vi "Filter Get Mode.vi"(11 "mode":u32) -> (2 "function return":u32, 3 "mode out":u32)   [LabVIEW 2018, in "AndorSDK.lvlib"]
doc: "EXPNETTYPE unsigned int WINAPI Filter_GetMode(unsigned int * mode);"
uses:
  AndorSDK.lvlib
  ATMCD32D.dll
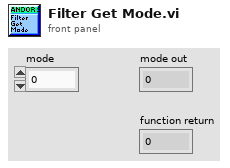
[diagram p1: front panel]
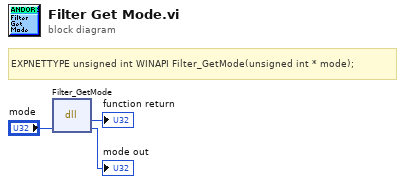
[diagram p0: block diagram]
diagram:
  # "EXPNETTYPE unsigned int WINAPI Filter_GetMode(unsigned int * mode);"
  n1 = dll-call lib="PTH2babs E\nPersönliches02 - Arbeit03-HiwijobsLabviewCodelibANDOR\tAndor SDK\nATMCD32D.*" fn="Filter_GetMode"("mode"="mode") -> (→"function return":u32, "mode"=→"mode out":u32)  [unwired: 3 in, 2 out]
